vi "start.vi"(8 "error in (no error)":errorcluster, 11 "Model in":refnum<class "Model.lvclass">) -> (0 "error out":errorcluster, 3 "Model out":refnum<class "Model.lvclass">)   [LabVIEW 2013, in "Model.lvclass"]
uses:
  Model.lvclass
  Model.lvclass/Model.ctl
  <userlib>/Common/ILC/ILC/ILC.lvclass
  <userlib>/Common/Component/Application/Application/Application.lvclass
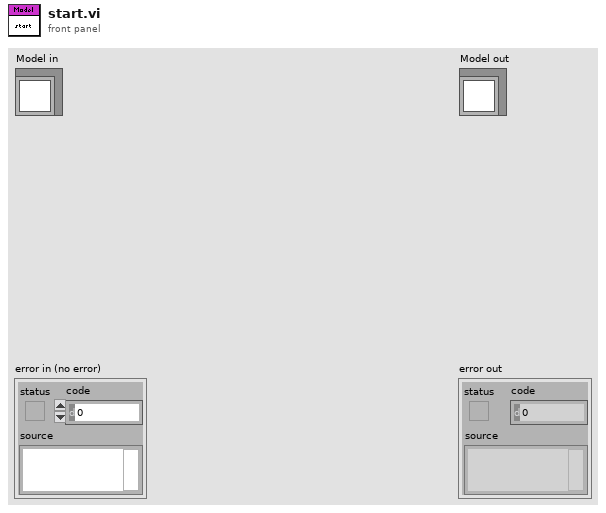
[diagram p1: front panel]
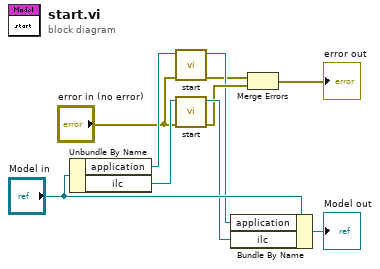
[diagram p0: block diagram]
diagram:
  n1 = Unbundle By Name("Model in") -> ("application"=w4:refnum<class "Application.lvclass">, "ilc"=w8:refnum<class "ILC.lvclass">)
  n2 = call <userlib>:"start.vi"("error in (no error)"="error in (no error)", "Application in"=w4) -> ("error out"=w2:errorcluster, "Application out"=w3:refnum<class "Application.lvclass">)  [unwired: 8 in]
  n3 = call <userlib>:"start.vi"("error in (no error)"="error in (no error)", "ILC in"=w8) -> ("error out"=w6:errorcluster, "ILC out"=w7:refnum<class "ILC.lvclass">)  [unwired: 8 in]
  n4 = Bundle By Name(cluster="Model in", "application"=w3, "ilc"=w7) -> (→"Model out":refnum<class "Model.lvclass">)
  n5 = Merge Errors(w2, w6) -> (→"error out":errorcluster)
